vi "Update 1 Cart Status.vi"(5 "Selection":T1, 7 "FP":T2, 8 "error in (no error)":errorcluster, 9 "String":string, 10 "Cartridge":i32) -> (0 "error out":errorcluster)   [LabVIEW 2018]
uses:
  Main Refs.ctl
  Hardware/Tecan/Pump Config.ctl
  Vacuum Specs.ctl
  Timing Specs.ctl
  Cartridges.ctl
  Cartridge Status.ctl
  Commands.ctl
  Lib/Time/Wells.ctl
  Lib/Time/Bottles.ctl
  Process State.ctl
  Vacuum Test.ctl
  Update Single Cart.ctl
panel:
  # "Tecan Pump"
  # "Vacuum"
  # "General"
  # "Timing"
  # "Protocol"
  # "Zaber"
  # "NFC Reader 1"
  # "NFC  Reader 2"
  # "NFC Reader 3"
  # "NFC Reader 4"
  # "System"
  # "Cartridge Utitlies"
  # "Wells"
  # "times"
  # "from"
  # "State Machine"
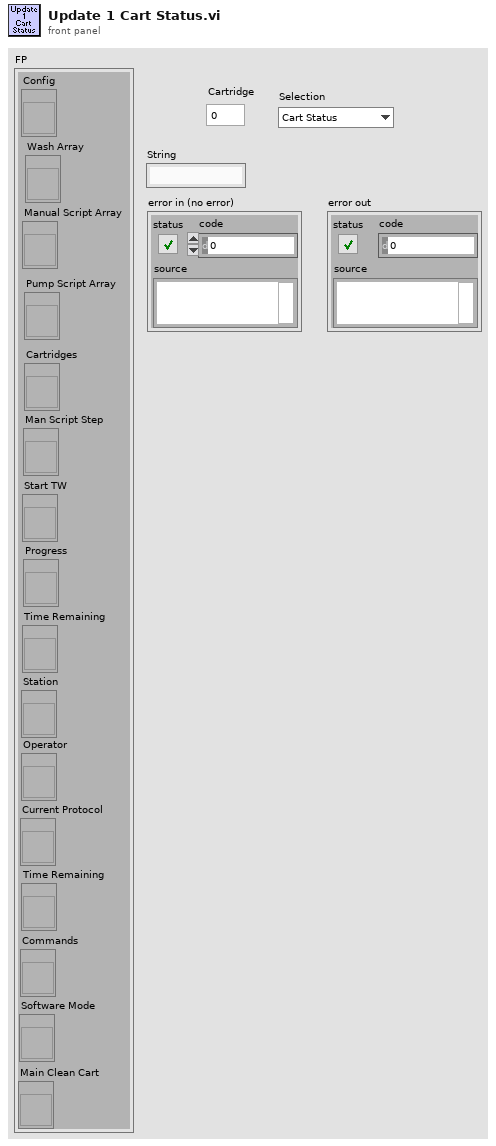
[diagram p1: front panel]
types:
  T1 = typedef "Update Single Cart.ctl" = enum16{"Cart Status", "Cart Reagent"}
  T2 = typedef "Main Refs.ctl" = cluster{"Config":refnum<vi>, "Wash Array":refnum<vi>, "Manual Script Array":refnum<vi>, "Pump Script Array":refnum<vi>, "Cartridges":refnum<vi>, "Man Script Step":refnum<vi>, "Start TW":refnum<vi>, "Progress":refnum<vi>, "Time Remaining":refnum<vi>, "Station":refnum<vi>, "Operator":refnum<vi>, "Current Protocol":refnum<vi>, "Time Remaining":refnum<vi>, "Commands":refnum<vi>, "Software Mode":refnum<vi>, "Main Clean Cart":refnum<vi>}
  T3 = typedef "Cartridges.ctl" = cluster{"Cartridge 1":T4, "Cartridge 2":T4, "Cartridge 3":T4, "Cartridge 4":T4, "Current Status":string}
  T4 = typedef "Cartridge Status.ctl" = cluster{"Serial Number":string, "Reagent":string, "Cart Status":string, "Inserted":bool, "Eject":bool}
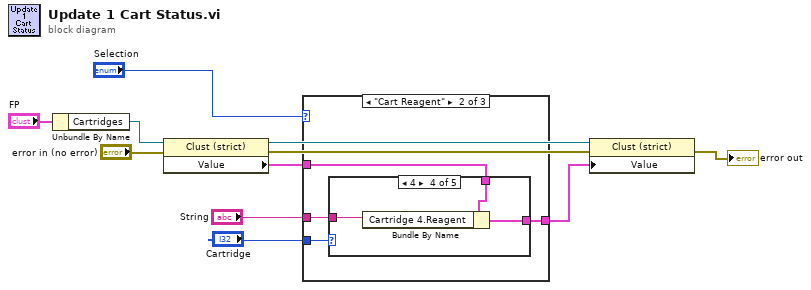
[diagram p0: block diagram]
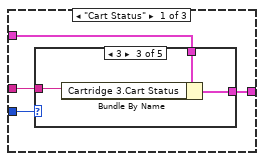
[diagram p2: hidden frame]
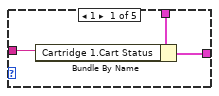
[diagram p3: hidden frame]
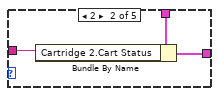
[diagram p4: hidden frame]
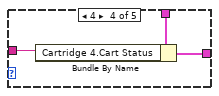
[diagram p5: hidden frame]
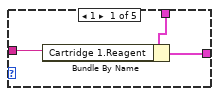
[diagram p7: hidden frame]
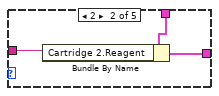
[diagram p8: hidden frame]
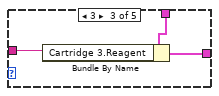
[diagram p9: hidden frame]
diagram:
  n1 = Unbundle By Name("FP") -> ("Cartridges"=w2:refnum<vi>)
  n2 = property class="Clust (strict)"(reference=w2, error in="error in (no error)") -> (reference out=w10:refnum<vi>, error out=w7:errorcluster, "Value"=w11:T3)
  n3 = case shown="\"Cart Reagent\"" "Selection" {
    tunnel: w11 -> [w15 w32 w46]
    tunnel: [w14 w31 w46] -> w9
    tunnel: "Cartridge" -> [w13 w30 _]
    tunnel: "String" -> [w12 w29 _]
    frame "Cart Status" {
      n4 = case shown="3" w13 {
        tunnel: w15 -> [w18 w21 w24 w27 w28]
        tunnel: [w17 w20 w23 w26 w28] -> w14
        tunnel: w12 -> [w16 w19 w22 w25 _]
        frame 1 {
          n5 = Bundle By Name(cluster=w18, "Cartridge 1.Cart Status"=w16) -> (w17:T3)
        }
        frame 2 {
          n6 = Bundle By Name(cluster=w21, "Cartridge 2.Cart Status"=w19) -> (w20:T3)
        }
        frame 3 {
          n7 = Bundle By Name(cluster=w24, "Cartridge 3.Cart Status"=w22) -> (w23:T3)
        }
        frame 4 {
          n8 = Bundle By Name(cluster=w27, "Cartridge 4.Cart Status"=w25) -> (w26:T3)
        }
        frame Default {
        }
      }
    }
    frame "Cart Reagent" {
      n9 = case shown="4" w30 {
        tunnel: w32 -> [w35 w38 w41 w44 w45]
        tunnel: [w34 w37 w40 w43 w45] -> w31
        tunnel: w29 -> [w33 w36 w39 w42 _]
        frame 1 {
          n10 = Bundle By Name(cluster=w35, "Cartridge 1.Reagent"=w33) -> (w34:T3)
        }
        frame 2 {
          n11 = Bundle By Name(cluster=w38, "Cartridge 2.Reagent"=w36) -> (w37:T3)
        }
        frame 3 {
          n12 = Bundle By Name(cluster=w41, "Cartridge 3.Reagent"=w39) -> (w40:T3)
        }
        frame 4 {
          n13 = Bundle By Name(cluster=w44, "Cartridge 4.Reagent"=w42) -> (w43:T3)
        }
        frame Default {
        }
      }
    }
    frame Default {
    }
  }
  n14 = property class="Clust (strict)"(reference=w10, error in=w7, "Value"=w9) -> (error out=→"error out":errorcluster)  [unwired: 1 out]
